vi "Set Defer Updates.vi"(8 "error in (no error)":errorcluster, 10 "Defer Updates":bool, 11 "PanelArray in":refnum<class "PanelArray.lvclass">) -> (0 "error out":errorcluster, 3 "PanelArray out":refnum<class "PanelArray.lvclass">)   [LabVIEW 2018, in "OOPanel.lvlib" / "PanelArray.lvclass"]
uses:
  PanelArray.lvclass
  PanelArray.lvclass/PanelArray.ctl
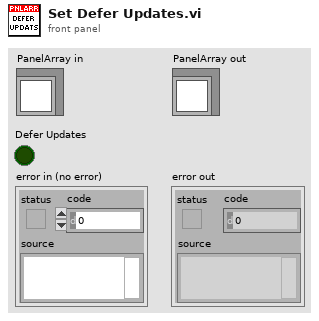
[diagram p1: front panel]
types:
  T1 = typedef "OOPanel.lvlib/PanelArray.lvclass/Ref Data.ctl" = cluster{"State":T2, "Refs":T3, "Events":T4, "Scrolling":T5, "Panels":T6}
  T2 = typedef "OOPanel.lvlib/PanelArray.lvclass/State.ctl" = cluster{"Defer Updates":bool, "Running":bool, "Dynamic Sizing":bool, "Borders":bool}
  T3 = typedef "OOPanel.lvlib/PanelArray.lvclass/Refs.ctl" = cluster{"SubPanels":refnum<vi>[], "Scrollbar":refnum<vi>, "Owning Panel":refnum<vi>}
  T4 = typedef "OOPanel.lvlib/PanelArray.lvclass/Events.ctl" = cluster{"Close":refnum<user-event>}
  T5 = typedef "OOPanel.lvlib/PanelArray.lvclass/Scrolling.ctl" = cluster{"Size":i32, "Max":i32, "Current":i32, "Top Index":i32, "Heights":i32[]}
  T6 = typedef "OOPanel.lvlib/PanelArray.lvclass/Panels.ctl" = cluster{"All":refnum<class "Panel.lvclass">[], "Visible":refnum<class "Panel.lvclass">[], "Blank":refnum<class "ArrayBlank.lvclass">}
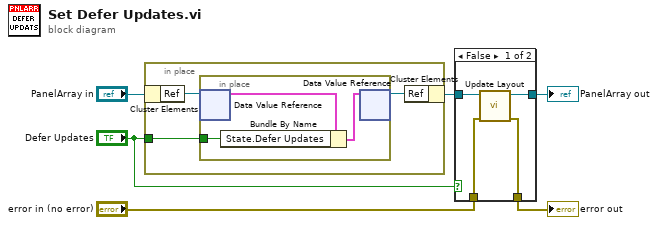
[diagram p0: block diagram]
diagram:
  n1 = in-place {
    in-place-border: "Defer Updates" -> [w9]
    n2 = in-place-cluster #1("PanelArray in") -> ("Ref"=w8:refnum<data-value>)
    n3 = in-place {
      in-place-border: w9 -> [w11]
      n4 = in-place-dvr #2(w8) -> (w12:T1)  [unwired: 1 out]
      n5 = Bundle By Name(cluster=w12, "State.Defer Updates"=w11) -> (w10:T1)
      n6 = in-place-dvr #2(w10) -> (w7:refnum<data-value>)  [unwired: 1 out]
    }
    n7 = in-place-cluster #1("Ref"=w7) -> (w5:refnum<class "PanelArray.lvclass">)
  }
  n8 = case shown="False" "Defer Updates" {
    tunnel: w5 -> [w16 w18]
    tunnel: [w15 w18] -> w4
    tunnel: "error in (no error)" -> [w14 w17]
    tunnel: [w13 w17] -> w1
    frame False {
      n9 = call "Update Layout.vi"("error in (no error)"=w14, "PanelArray in"=w16) -> ("error out"=w13:errorcluster, "PanelArray out"=w15:refnum<class "PanelArray.lvclass">)  [unwired: 8 in]
    }
    frame True {
    }
  }
  "error out" <- w1
  "PanelArray out" <- w4
